vi "Lex Nothing.vi"(8 "Error In":errorcluster) -> (0 "Error Out":errorcluster)   [LabVIEW 2018, in "Tests.lvlib" / "Lexer.lvlib"]
uses:
  Lexer.lvlib
  src/Toolkit/Low-Level/Support/Lex String.vi
  <vilib>/addons/_JKI Toolkits/Caraya/classes/Test/Test.lvclass
  <vilib>/addons/_JKI Toolkits/Caraya/classes/Assert/Assert.lvclass
  src/Toolkit/Toolkit.lvlib
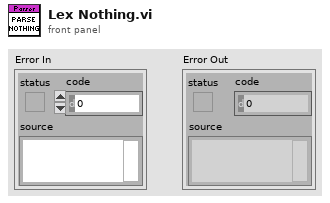
[diagram p1: front panel]
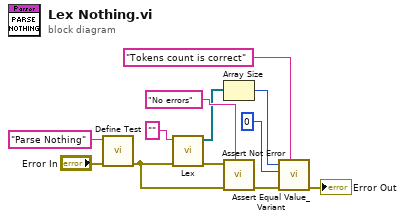
[diagram p0: block diagram]
diagram:
  n1 = call <vilib>:"Define Test.vi"("error in (no error)"="Error In", "Label (VI Title)"="Parse Nothing") -> ("error out"=w2:errorcluster)  [unwired: 9 in]
  n2 = call-poly "Lex.vi"("Error In"=w2, "Input"="" ("String")) -> ("Error Out"=w10:errorcluster, "Tokens"=w5:refnum<class "Abstract.lvclass">[])  [unwired: 8 in]
  n3 = Array Size(array=w5) -> (size(s)=w4:i32)
  n4 = call <vilib>:"Assert Not Error.vi"("Label"="No errors", "error in (no error)"=w2, "Not Error?"=w10) -> ("error out"=w9:errorcluster)  [unwired: 8 in]
  n5 = call <vilib>:"Assert Equal Value_Variant.vi"("Label"="Tokens count is correct", "error in (no error)"=w9, "Y"=0 ("size(s)"), "X"=w4) -> ("error out"=→"Error Out":errorcluster)  [unwired: 7 in]
